vi "testRPM2.vi"() -> ()   [LabVIEW 2014]
uses:
  <vilib>/Analysis/baseanly.llb/Mean (DBL).vi
  <vilib>/Analysis/NI_AALBase.lvlib
panel:
  out "Filtered Signal 3":dynamicdata(graph) caption="Filtered Signal"
  in  "Low Base speed":dbl
  in  "Fator":dbl
  out "Velocidade(km_h)":dbl
  out "RPM":dbl
  out "Frequency (RPM)":dbl
  out "Filtered Signal 2":dynamicdata(graph) caption="Filtered Signal"
  out "error out":errorcluster
  in  "stop":bool
  out "Frequency":dbl
  out "Raw Signal":dynamicdata(graph) caption="Filtered Signal"
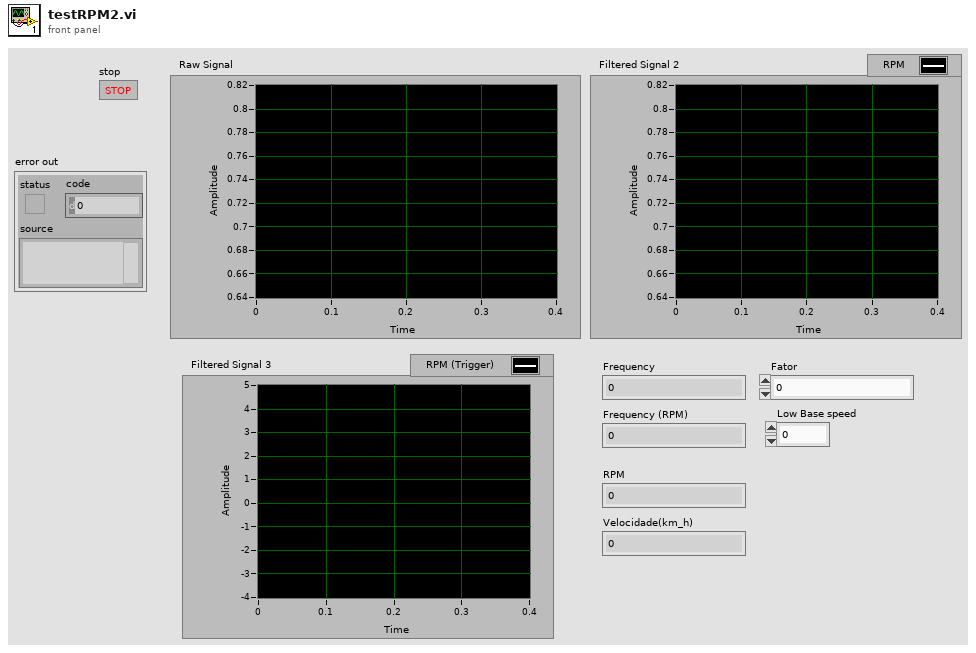
[diagram p1: front panel]
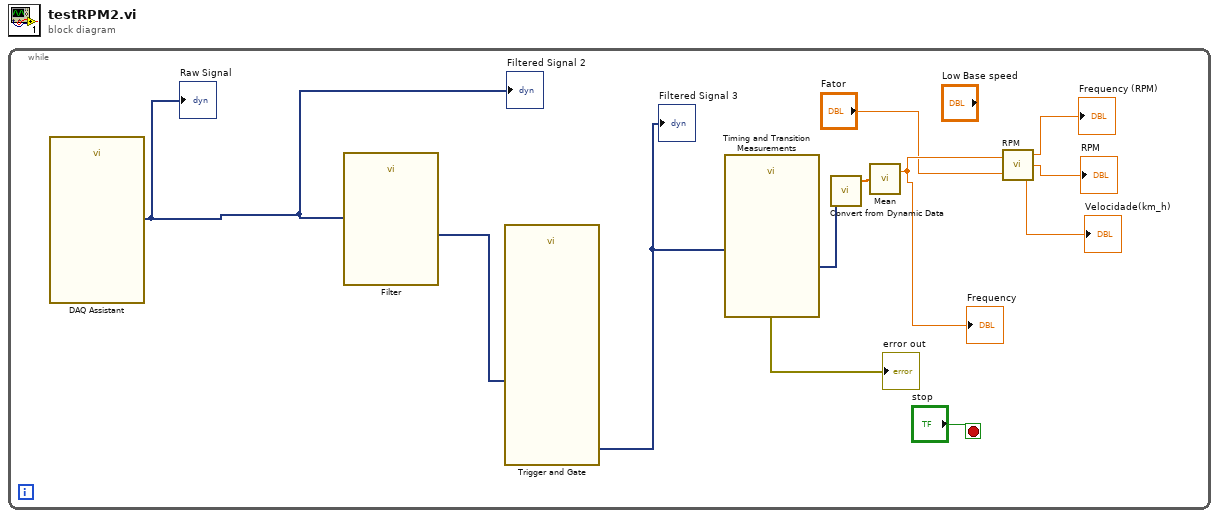
[diagram p0: block diagram]
diagram:
  n1 = while {
    stop <- "stop" stop-if-true
    n2 = call "DAQ Assistant"() -> ("data"=w3:dynamicdata)  [unwired: 16 in, 3 out]
    "Raw Signal" <- w3
    "Filtered Signal 2" <- w3
    n3 = call "Filter"("Signal"=w3) -> ("Filtered Signal"=w2:dynamicdata)  [unwired: 9 in, 1 out]
    n4 = call "Trigger and Gate"("Signals"=w2) -> ("Triggered Signals"=w1:dynamicdata)  [unwired: 7 in, 3 out]
    "Filtered Signal 3" <- w1
    n5 = call "Timing and Transition Measurements"("Signals"=w1) -> ("error out"=→"error out":errorcluster, "Frequency"=w10:dynamicdata)  [unwired: 9 in]
    n6 = call "Convert from Dynamic Data"("Dynamic Data Type"=w10) -> ("Array"=w9:dbl[])  [unwired: 3 in]
    n7 = call-poly <vilib>:"Mean.vi"("X"=w9) -> ("mean"=w5:dbl)  [unwired: 1 out]
    "Frequency" <- w5
    n8 = call "RPM.vi"("data"=w5, "factor"="Fator") -> ("Frequency"=→"Frequency (RPM)":dbl, "RPM"=→"RPM":dbl, "km/h"=→"Velocidade(km_h)":dbl)
  }
